vi "PCSMain.panel.vi"(0 "object ref":refnum<vi>, 5 "error in (no error)":errorcluster) -> (19 "error out":errorcluster)   [LabVIEW 2014, in "PCSMain.lvlib"]
doc: "This is just an example for a GUI thread.\n\nLicense Agreement for this software:\n\nCopyright (C)\nGesellschaft für Schwerionenforschung, GSI\nPlanckstr. 1\n64291 Darmstadt\nGermany\n\nContact: D.Beck@gsi.de \n\nThis program is free software; you can redistribute it and/or modify it under the terms of the GNU General Public License as published by the Free Software Foundation; either version 2 of the license, or (at your option) any later version.\n\nThis program is distributed in the hope that it will be useful, but WITHOUT ANYW ARRANTY; without even the implied warranty of MERCHANTABILITY or FITNESS FOR A PARTICULAR PURPOSE. See the GNU General License for more details (http://www.gnu.org).\n\nGesellschaft für Schwerionenforschung, GSI\nPlanckstr. 1, 64291 Darmstadt, Germany\nFor all questions and ideas contact: M.Richter@gsi.de, H.Brand@gsi.de or D.Beck@gsi.de.\nLast update: 18-DEC-2002"
uses:
  PCSMain.lvlib
  CSCore/CSObj/CSObj.lvlib
  PH_Common/PH_Common.lvlib
panel:
  in  "VISA":bool
  in  "Powermeter Statistician":bool
  in  "Powermeter List":bool
  in  "SHS Anal Statistician":bool
  in  "SHS Analyzer":bool
  in  "SHS Analysis Calibrator":bool
  in  "Remote Desktop Connection":bool
  in  "Minimize":bool
  in  "Beckhoff Watch Dog":bool
  in  "Countdown":bool
  in  "Seq Watch":bool
  in  "Vacuum Controllers":bool
  in  "SSAC":bool
  in  "Switch List":bool
  in  "BB List":bool
  in  "Spectrometer":bool
  in  "Z6 Beamline":bool
  in  "6P List":bool
  in  "Scopes":bool
  in  "Current Meas":bool
  in  "Calorimeter":bool
  in  "Cam List":bool
  in  "PCS System Indicator":bool caption="PCS"
  in  "Fast CoG":bool
  in  "Image Statistician":bool
  in  "Powermeter":bool
  in  "DataViewer":bool
  in  "Beamline":bool
  out "stopped":bool
  in  "BlackBoxes":bool
  in  "Operators":bool
  in  "Calibrator":bool
  in  "GateDelayGens":bool
  in  "Switch GUIs":bool
  in  "Motion GUIs":bool
  in  "Cameras":bool
  in  "Sequencer":bool
  in  "Delete":bool
  out "loop counter":i32
  # "PCS"
  # "3.40"
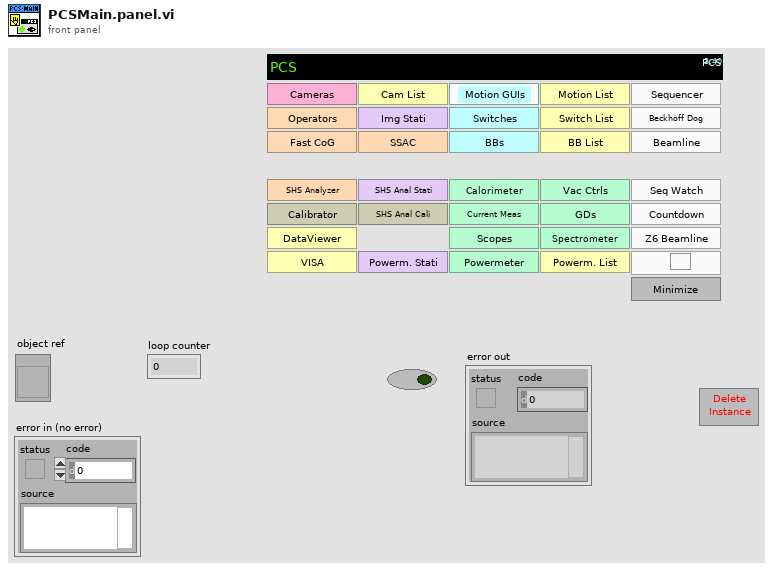
[diagram p1: front panel]
types:
  T1 = enum16{"None", "PCS Main", "Z6 Main", "PCS Beamline", "Z6 Beamline", "Image Statistician", "Powermeter Statistician", "SHS Anal Statistician", "Image Center of Gravity", "Image Calibrator", "SHS Analysis Calibrator"}
  T2 = enum16{"None", "PCS Main", "Z6 Main", "PCS Beamline", "Z6 Beamline", "Image Statistician", "Powermeter Statistician", "SHS Anal Statistician", "Image Center of Gravity", "Image Calibrator", "SHS Analysis Calibrator", "Cam List", "Powermeterlist", "6P List", "BB List", "Switch List", "Sequence Watch"}
  T3 = typedef "PCSMain.lvlib/PCSMain.i attribute.ctl" = cluster{"System Objects":cluster{"Spectrometer Objects":string[], "Camera Objects":string[], "Image Operator Objects":string[], "Gate- and Delaygenerators":string[], "Current Meas Objects":string[], "Calorimeter Objects":string[], "Powermeter Objects":string[], "SSAC Objects":string[], "Vacuum Control Objects":string[], "Countdown Counter Objects":string[], "Beckhoff Watchdog Objects":string[], "SHS Analyzer Objects":string[]}, "Local Objects":cluster{"Spectrometer Objects":string[], "Camera Objects":string[], "Image Operator Objects":string[], "Gate- and Delaygenerators":string[], "Current Meas Objects":string[], "Calorimeter Objects":string[], "Powermeter Objects":string[], "SSAC Objects":string[], "Vacuum Control Objects":string[], "Countdown Counter Objects":string[], "Beckhoff Watchdog Objects":string[], "SHS Analyzer Objects":string[]}, "Systems on same node":string[], "Data Viewer visible?":bool, "Running Objects":cluster{"Operators":bool, "SHS Analyzers":bool}, "Cam Instance System ID":string, "Black Box Objects":string[], "Switch Objects":string[], "Motion GUI Objects":string[], "Osci Objects":string[]}
  T4 = enum16{"PCS", "Laser", "Vision", "PP", "Special", "Beckhoff"}
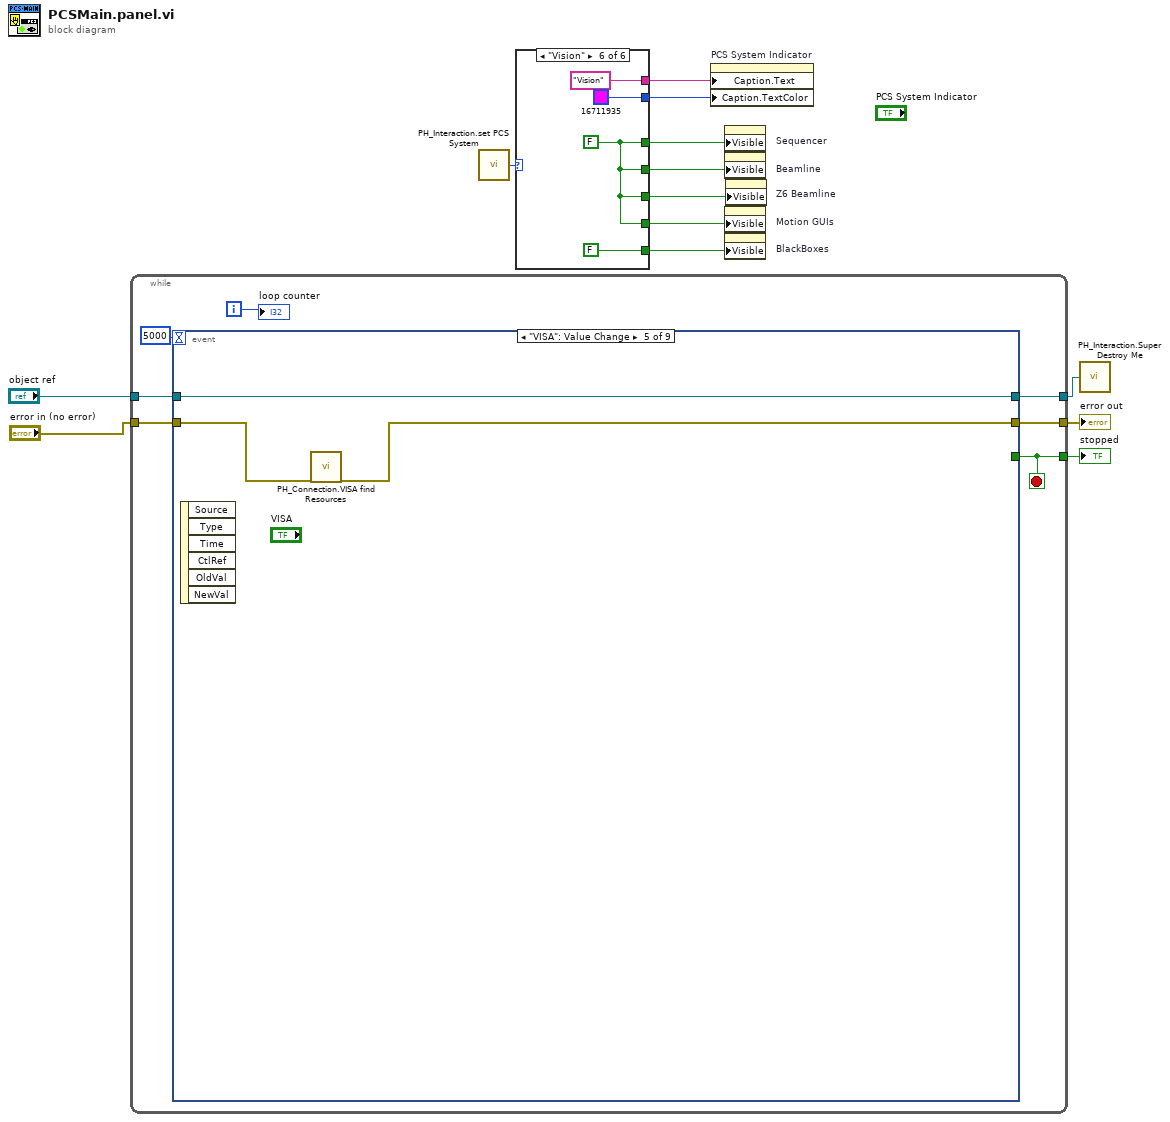
[diagram p0: block diagram]
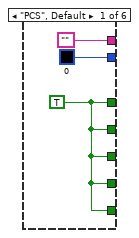
[diagram p2: hidden frame]
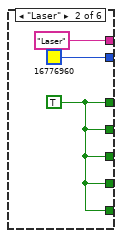
[diagram p3: hidden frame]
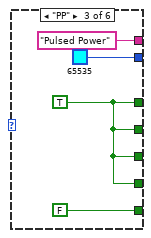
[diagram p4: hidden frame]
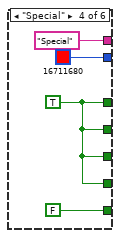
[diagram p5: hidden frame]
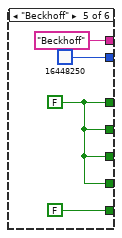
[diagram p6: hidden frame]
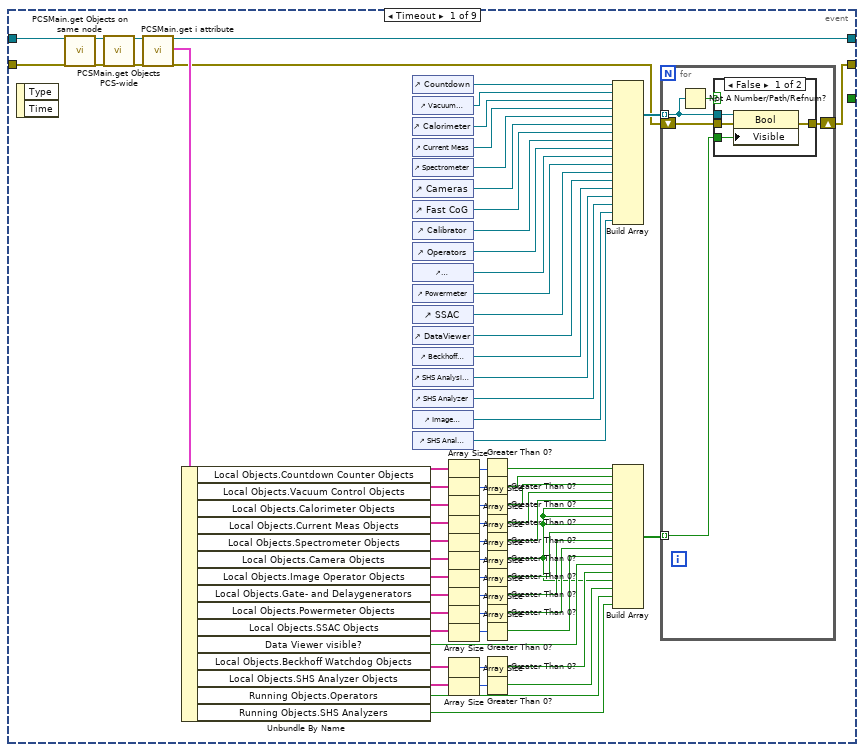
[diagram p7: hidden frame]
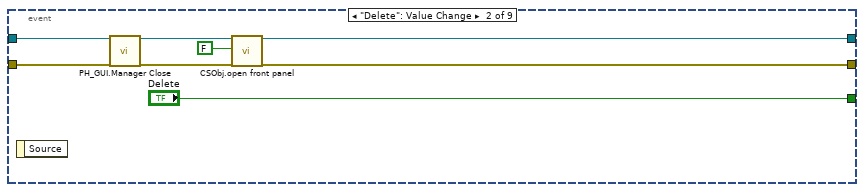
[diagram p9: hidden frame]
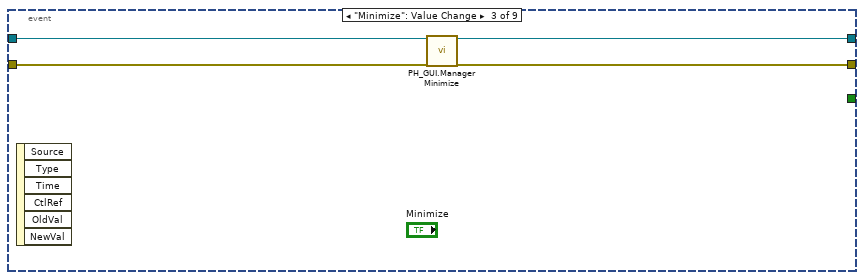
[diagram p10: hidden frame]
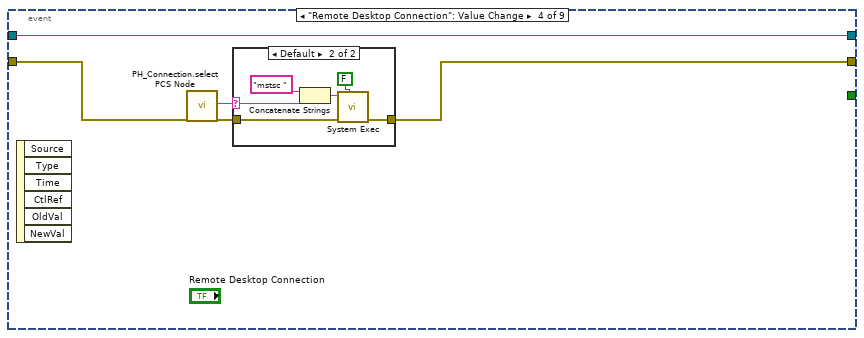
[diagram p11: hidden frame]
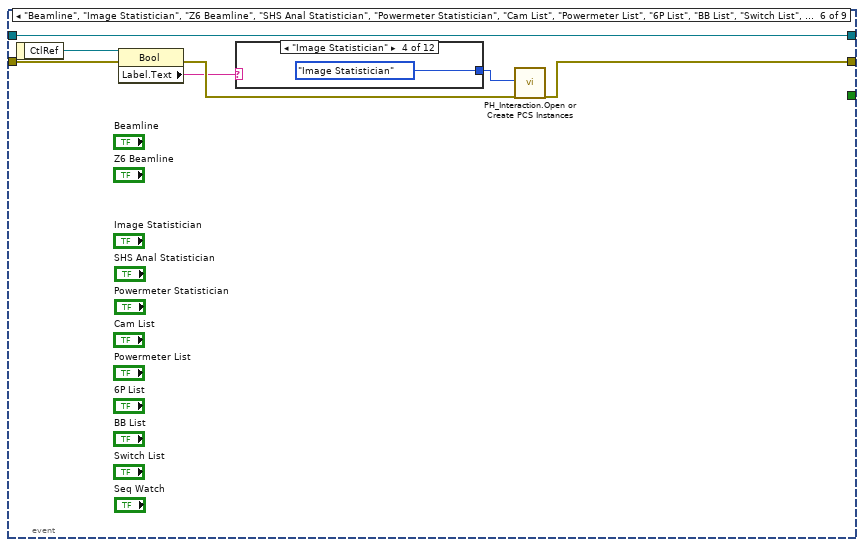
[diagram p13: hidden frame]
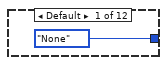
[diagram p14: hidden frame]
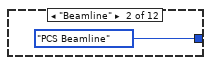
[diagram p15: hidden frame]
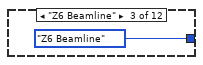
[diagram p16: hidden frame]
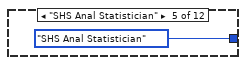
[diagram p17: hidden frame]
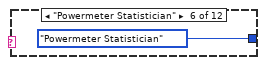
[diagram p18: hidden frame]
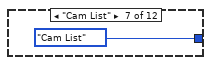
[diagram p19: hidden frame]
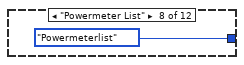
[diagram p20: hidden frame]
diagram:
  n1 = while {
    tunnel: "object ref" -> [w16]
    tunnel: [w15] -> w11
    tunnel: [w19] -> w12
    tunnel: "error in (no error)" -> [w18]
    tunnel: [w17] -> w13
    i -> [w20]
    stop <- w17 stop-if-true
    n2 = event shown="[4] \"VISA\": Value Change" {
      selector: _ -> [_ _ _ _ _ _ _ _ _]
      dyn-events: _ -> [_ _ _ _ _ _ _ _ _]
      timeout: 5000 -> [_ _ _ _ _ _ _ _ _]
      tunnel: w16 -> [w88 w105 w111 w115 w126 w130 w151 w171 w236]
      tunnel: [_ "Delete" _ _ _ _ _ _ _] -> w17
      tunnel: [w63 w104 w108 w113 w124 w133 w156 w169 w234] -> w19
      tunnel: w18 -> [w89 w101 w110 w116 w125 w131 w154 w170 w233]
      tunnel: [w62 w103 w109 w115 w126 w130 w150 w161 w235] -> w15
      event Timeout {
        n3 = event-data() -> ()  [unwired: 1 in, 2 out]
        n4 = call "PCSMain.get Objects on same node.vi"("i ref in"=w88, "error in (no error)"=w89) -> ("i ref out"=w24:refnum<vi>, "error out"=w22:errorcluster)  [unwired: 16 in]
        n5 = call "PCSMain.get Objects PCS-wide.vi"("i ref in"=w24, "error in (no error)"=w22) -> ("i ref out"=w23:refnum<vi>, "error out"=w21:errorcluster)  [unwired: 16 in]
        n6 = call "PCSMain.get i attribute.vi"("i ref in"=w23, "error in (no error)"=w21) -> ("i ref out"=w62:refnum<vi>, "i attribute"=w87:T3, "error out"=w64:errorcluster)  [unwired: 15 in]
        n7 = Unbundle By Name(w87) -> ("Local Objects.Countdown Counter Objects"=w44:string[], "Local Objects.Vacuum Control Objects"=w48:string[], "Local Objects.Calorimeter Objects"=w83:string[], "Local Objects.Current Meas Objects"=w76:string[], "Local Objects.Spectrometer Objects"=w74:string[], "Local Objects.Camera Objects"=w72:string[], "Local Objects.Image Operator Objects"=w71:string[], "Local Objects.Gate- and Delaygenerators"=w69:string[], "Local Objects.Powermeter Objects"=w67:string[], "Local Objects.SSAC Objects"=w39:string[], "Data Viewer visible?"=w50:bool, "Local Objects.Beckhoff Watchdog Objects"=w41:string[], "Local Objects.SHS Analyzer Objects"=w31:string[], "Running Objects.Operators"=w26:bool, "Running Objects.SHS Analyzers"=w25:bool)
        n8 = control-ref of="Countdown"() -> (w45:refnum<vi>)
        n9 = control-ref of="Vacuum Controllers"() -> (w49:refnum<vi>)
        n10 = control-ref of="Calorimeter"() -> (w61:refnum<vi>)
        n11 = control-ref of="Current Meas"() -> (w60:refnum<vi>)
        n12 = control-ref of="Spectrometer"() -> (w59:refnum<vi>)
        n13 = control-ref of="Cameras"() -> (w58:refnum<vi>)
        n14 = control-ref of="Fast CoG"() -> (w54:refnum<vi>)
        n15 = control-ref of="Calibrator"() -> (w53:refnum<vi>)
        n16 = control-ref of="Operators"() -> (w57:refnum<vi>)
        n17 = control-ref of="GateDelayGens"() -> (w56:refnum<vi>)
        n18 = control-ref of="Powermeter"() -> (w55:refnum<vi>)
        n19 = control-ref of="SSAC"() -> (w52:refnum<vi>)
        n20 = control-ref of="DataViewer"() -> (w51:refnum<vi>)
        n21 = control-ref of="Beckhoff Watch Dog"() -> (w36:refnum<vi>)
        n22 = control-ref of="SHS Analysis Calibrator"() -> (w34:refnum<vi>)
        n23 = control-ref of="SHS Analyzer"() -> (w29:refnum<vi>)
        n24 = control-ref of="Image Statistician"() -> (w28:refnum<vi>)
        n25 = control-ref of="SHS Anal Statistician"() -> (w27:refnum<vi>)
        n26 = Array Size(array=w44) -> (size(s)=w42:i32)
        n27 = Array Size(array=w48) -> (size(s)=w46:i32)
        n28 = Array Size(array=w83) -> (size(s)=w84:i32)
        n29 = Array Size(array=w76) -> (size(s)=w81:i32)
        n30 = Array Size(array=w74) -> (size(s)=w80:i32)
        n31 = Array Size(array=w72) -> (size(s)=w79:i32)
        n32 = Array Size(array=w71) -> (size(s)=w78:i32)
        n33 = Array Size(array=w69) -> (size(s)=w77:i32)
        n34 = Array Size(array=w67) -> (size(s)=w65:i32)
        n35 = Array Size(array=w39) -> (size(s)=w38:i32)
        n36 = Array Size(array=w41) -> (size(s)=w40:i32)
        n37 = Array Size(array=w31) -> (size(s)=w32:i32)
        n38 = Greater Than 0?(x=w42) -> (x > 0?=w43:bool)
        n39 = Greater Than 0?(x=w46) -> (x > 0?=w47:bool)
        n40 = Greater Than 0?(x=w84) -> (x > 0?=w82:bool)
        n41 = Greater Than 0?(x=w81) -> (x > 0?=w75:bool)
        n42 = Greater Than 0?(x=w80) -> (x > 0?=w73:bool)
        n43 = Greater Than 0?(x=w79) -> (x > 0?=w33:bool)
        n44 = Greater Than 0?(x=w78) -> (x > 0?=w70:bool)
        n45 = Greater Than 0?(x=w77) -> (x > 0?=w68:bool)
        n46 = Greater Than 0?(x=w65) -> (x > 0?=w66:bool)
        n47 = Greater Than 0?(x=w38) -> (x > 0?=w37:bool)
        n48 = Greater Than 0?(x=w40) -> (x > 0?=w35:bool)
        n49 = Greater Than 0?(x=w32) -> (x > 0?=w30:bool)
        n50 = Build Array(w45, w49, w61, w60, w59, w58, w54, w53, w57, w56, w55, w52, w51, w36, w34, w29, w28, w27) -> (w86:refnum<vi>[])
        n51 = Build Array(w43, w47, w82, w75, w73, w33, w33, w33, w70, w68, w66, w37, w50, w35, w33, w30, w26, w25) -> (w85:bool[])
        n52 = for {
          tunnel: w85 -> [w90] mode=indexing
          tunnel: w86 -> [w93] mode=indexing
          shift-right: [w92] -> w63
          shift-left: w64 -> [w91]
          n53 = Not A Number/Path/Refnum?(number/path/refnum=w93) -> (NaN/Path/Refnum?=w94:bool)
          n54 = case shown="False" w94 {
            tunnel: w90 -> [w98 _]
            tunnel: w93 -> [w97 _]
            tunnel: w91 -> [w96 w99]
            tunnel: [w95 w99] -> w92
            frame False {
              n55 = property class="Bool"(reference=w97, error in=w96, "Visible"=w98) -> (error out=w95:errorcluster)  [unwired: 1 out]
            }
            frame True {
            }
          }
        }
      }
      event "Delete": Value Change {
        n56 = event-data() -> ()  [unwired: 1 in, 1 out]
        n57 = call "PH_GUI.Manager Close.vi"("i ref in"=w105, "error in"=w101) -> ("i ref out"=w102:refnum<vi>, "error out"=w100:errorcluster)  [unwired: 16 in]
        n58 = call "CSObj.open front panel.vi"("i ref in"=w102, "frontPanelOpen"=FALSE ("front panel open"), "error in (no error)"=w100) -> ("i ref out"=w103:refnum<vi>, "error out"=w104:errorcluster)  [unwired: 15 in]
      }
      event "Minimize": Value Change {
        n59 = event-data() -> ()  [unwired: 1 in, 6 out]
        n60 = call "PH_GUI.Manager Minimize.vi"("i ref in"=w111, "error in"=w110) -> ("i ref out"=w109:refnum<vi>, "error out"=w108:errorcluster)  [unwired: 16 in]
      }
      event "Remote Desktop Connection": Value Change {
        n61 = event-data() -> ()  [unwired: 1 in, 6 out]
        n62 = call "PH_Connection.select PCS Node.vi"("error in"=w116) -> ("string out"=w112:string, "error out"=w114:errorcluster)  [unwired: 17 in]
        n63 = case shown="Default" w112 {
          selector: w112 -> [_ w118]
          tunnel: w114 -> [w117 w120]
          tunnel: [w117 w119] -> w113
          frame "", "N/A" {
          }
          frame Default {
            n64 = Concatenate Strings("mstsc " ("command line"), w118) -> (w122:string)
            n65 = call <vilib>:"System Exec.vi"("wait until completion? (T)"=FALSE, "error in (no error)"=w120, "command line"=w122) -> ("error out"=w119:errorcluster)  [unwired: 5 in, 3 out]
          }
        }
      }
      event "VISA": Value Change {
        n66 = event-data() -> ()  [unwired: 1 in, 6 out]
        n67 = call "PH_Connection.VISA find Resources.vi"("error in"=w125) -> ("error out"=w124:errorcluster)  [unwired: 17 in, 1 out]
      }
      event "Beamline", "Image Statistician", "Z6 Beamline", "SHS Anal Statistician", "Powermeter Statistician", "Cam List", "Powermeter List", "6P List", "BB List", "Switch List", "Seq Watch": Value Change {
        n68 = event-data() -> ("CtlRef"=w132:refnum<vi>)  [unwired: 1 in]
        n69 = property class="Bool"(reference=w132, error in=w131) -> (error out=w129:errorcluster, "Label.Text"=w128:string)  [unwired: 1 out]
        n70 = case shown="\"Image Statistician\"" w128 {
          tunnel: [T1."None" ("Instance to create or open") T1."PCS Beamline" ("Instance to create or open") T1."Z6 Beamline" ("Instance to create or open") T1."Image Statistician" ("Instance to create or open") T1."SHS Anal Statistician" ("Instance to create or open") T1."Powermeter Statistician" ("Instance to create or open") T2."Cam List" ("Instance to create or open") T2."Powermeterlist" ("Instance to create or open") T2."6P List" ("Instance to create or open") T2."BB List" ("Instance to create or open") T2."Switch List" ("Instance to create or open") T2."Sequence Watch" ("Instance to create or open")] -> w127
          frame Default {
          }
          frame "Beamline" {
          }
          frame "Z6 Beamline" {
          }
          frame "Image Statistician" {
          }
          frame "SHS Anal Statistician" {
          }
          frame "Powermeter Statistician" {
          }
          frame "Cam List" {
          }
          frame "Powermeter List" {
          }
          frame "6P List" {
          }
          frame "BB List" {
          }
          frame "Switch List" {
          }
          frame "Seq Watch" {
          }
        }
        n71 = call "PH_Interaction.Open or Create PCS Instances.vi"("Instance to create or open"=w127, "error IO"=w129) -> ("error out"=w133:errorcluster)  [unwired: 17 in]
      }
      event "Calibrator", "SHS Analysis Calibrator", "Fast CoG": Value Change {
        n72 = event-data() -> ("CtlRef"=w155:refnum<vi>)  [unwired: 1 in]
        n73 = property class="Bool"(reference=w155, error in=w154) -> (error out=w153:errorcluster, "Label.Text"=w146:string)  [unwired: 1 out]
        n74 = call "PCSMain.get i attribute.vi"("i ref in"=w151, "error in (no error)"=w153) -> ("i ref out"=w150:refnum<vi>, "i attribute"=w149:T3, "error out"=w152:errorcluster)  [unwired: 15 in]
        n75 = case shown="\"SHS Analysis Calibrator\"" w146 {
          tunnel: [T1."None" ("Instance to create or open") T1."Image Calibrator" ("Instance to create or open") T1."SHS Analysis Calibrator" ("Instance to create or open") T1."Image Center of Gravity" ("Instance to create or open")] -> w147
          frame Default {
          }
          frame "Calibrator" {
          }
          frame "SHS Analysis Calibrator" {
          }
          frame "Fast CoG" {
          }
        }
        n76 = Unbundle By Name(w149) -> ("Cam Instance System ID"=w148:string)
        n77 = call "PH_Interaction.Open or Create PCS Instances.vi"("System ID (N/A)"=w148, "Instance to create or open"=w147, "error IO"=w152) -> ("error out"=w156:errorcluster)  [unwired: 16 in]
      }
      event "Spectrometer", "Cameras", "Operators", "GateDelayGens", "Current Meas", "Calorimeter", "Powermeter", "SSAC", "Vacuum Controllers", "Beckhoff Watch Dog", "SHS Analyzer", "Switch GUIs", "BlackBoxes", "Motion GUIs", "Scopes": Value Change {
        n78 = event-data() -> ("CtlRef"=w167:refnum<vi>)  [unwired: 1 in]
        n79 = property class="Bool"(reference=w167) -> ("Label.Text"=w165:string)  [unwired: 1 in, 2 out]
        n80 = call "PCSMain.get i attribute.vi"("i ref in"=w171, "error in (no error)"=w170) -> ("i ref out"=w162:refnum<vi>, "i attribute"=w166:T3, "error out"=w168:errorcluster)  [unwired: 15 in]
        n81 = case shown="\"Spectrometer\"" w165 {
          tunnel: w166 -> [_ w179 w182 w185 w188 w191 w194 w197 w200 w203 w206 w209 w212 w215 w218 w221]
          tunnel: [string[] [] ("Spectrometer Objects") w178 w180 w183 w186 w189 w193 w196 w199 w202 w205 w208 w211 w214 w217 w220] -> w163
          tunnel: ["N/A" ("Caption.Text") "Spectrometer" ("Caption.Text") "Switch GUIs" ("Caption.Text") "Black Boxes" ("Caption.Text") "Motion GUIs" ("Caption.Text") "Oscilloscopes" ("Caption.Text") "Cameras" ("Caption.Text") "Image Operators" ("Caption.Text") "SHS Analyzers" ("Caption.Text") "Gate and Delay Generators" ("Caption.Text") "Current Measurement" ("Caption.Text") "Calorimeter" ("Caption.Text") "Powermeter" ("Caption.Text") "SSAC" ("Caption.Text") "Vacuum Controller" ("Caption.Text") "Beckhoff Watchdog" ("Caption.Text")] -> w164
          frame Default {
          }
          frame "Spectrometer" {
            n82 = Unbundle By Name(w179) -> ("Local Objects.Spectrometer Objects"=w178:string[])
          }
          frame "Switch GUIs" {
            n83 = Unbundle By Name(w182) -> ("Switch Objects"=w180:string[])
          }
          frame "BlackBoxes" {
            n84 = Unbundle By Name(w185) -> ("Black Box Objects"=w183:string[])
          }
          frame "Motion GUIs" {
            n85 = Unbundle By Name(w188) -> ("Motion GUI Objects"=w186:string[])
          }
          frame "Scopes" {
            n86 = Unbundle By Name(w191) -> ("Osci Objects"=w189:string[])
          }
          frame "Cameras" {
            n87 = Unbundle By Name(w194) -> ("Local Objects.Camera Objects"=w193:string[])
          }
          frame "Operators" {
            n88 = Unbundle By Name(w197) -> ("Local Objects.Image Operator Objects"=w196:string[])
          }
          frame "SHS Analyzer" {
            n89 = Unbundle By Name(w200) -> ("Local Objects.SHS Analyzer Objects"=w199:string[])
          }
          frame "GateDelayGens" {
            n90 = Unbundle By Name(w203) -> ("Local Objects.Gate- and Delaygenerators"=w202:string[])
          }
          frame "Current Meas" {
            n91 = Unbundle By Name(w206) -> ("Local Objects.Current Meas Objects"=w205:string[])
          }
          frame "Calorimeter" {
            n92 = Unbundle By Name(w209) -> ("Local Objects.Calorimeter Objects"=w208:string[])
          }
          frame "Powermeter" {
            n93 = Unbundle By Name(w212) -> ("Local Objects.Powermeter Objects"=w211:string[])
          }
          frame "SSAC" {
            n94 = Unbundle By Name(w215) -> ("Local Objects.SSAC Objects"=w214:string[])
          }
          frame "Vacuum Controllers" {
            n95 = Unbundle By Name(w218) -> ("Local Objects.Vacuum Control Objects"=w217:string[])
          }
          frame "Beckhoff Watch Dog" {
            n96 = Unbundle By Name(w221) -> ("Local Objects.Beckhoff Watchdog Objects"=w220:string[])
          }
        }
        n97 = call "PH_Strings.select string from array.vi"("String Array in"=w163, "Caption.Text"=w164, "error in (no error)"=w168) -> ("string out"=w174:string, "index"=w172:i32, "error out"=w173:errorcluster)  [unwired: 14 in]
        n98 = case shown="Default" w172 {
          tunnel: w173 -> [w223 w228]
          tunnel: [w223 w227] -> w169
          tunnel: w174 -> [_ w226]
          tunnel: w162 -> [w222 w224]
          tunnel: [w222 w225] -> w161
          frame -1 {
          }
          frame Default {
            n99 = call "PH_Interaction.Open or Create Singleton Instance.vi"("i ref in"=w224, "Instance to create or to open"=w226, "error IO"=w228) -> ("i ref out"=w225:refnum<vi>, "error out"=w227:errorcluster)  [unwired: 15 in]
          }
        }
      }
      event "DataViewer", "Countdown", "Sequencer": Value Change {
        n100 = event-data() -> ("CtlRef"=w231:refnum<vi>)  [unwired: 1 in]
        n101 = property class="Bool"(reference=w231, error in=w233) -> (error out=w232:errorcluster, "Label.Text"=w230:string)  [unwired: 1 out]
        n102 = case shown="\"Countdown\"" w230 {
          tunnel: ["N/A" "Data_Viewer" "PHELIX_Sequencer_1" "Countdown"] -> w229
          frame Default {
          }
          frame "DataViewer" {
          }
          frame "Sequencer" {
          }
          frame "Countdown" {
          }
        }
        n103 = call "PH_Interaction.Open or Create Singleton Instance.vi"("i ref in"=w236, "Instance to create or to open"=w229, "error IO"=w232) -> ("i ref out"=w235:refnum<vi>, "error out"=w234:errorcluster)  [unwired: 15 in]
      }
    }
    "loop counter" <- w20
  }
  "error out" <- w12
  "stopped" <- w13
  n104 = call "PH_Interaction.set PCS System.vi"() -> ("Enum"=w10:T4)  [unwired: 1 in]
  n105 = case shown="\"Vision\"" w10 {
    tunnel: ["" "Laser" "Pulsed Power" "Special" "Beckhoff" "Vision"] -> w9
    tunnel: [w242 w245 w249 w253 w257 w261] -> w8
    tunnel: [w242 w245 w249 w253 w257 w261] -> w7
    tunnel: [w242 w245 w249 w253 w257 w261] -> w6
    tunnel: [w242 w245 FALSE FALSE FALSE FALSE] -> w5
    tunnel: [w242 w245 w249 w253 w257 w261] -> w4
    tunnel: [u32 0 ("Color Box") u32 16776960 ("Color Box") u32 65535 ("Color Box") u32 16711680 ("Color Box") u32 16448250 ("Color Box") u32 16711935 ("Color Box")] -> w1
    frame "PCS", Default {
      w242 = TRUE
    }
    frame "Laser" {
      w245 = TRUE
    }
    frame "PP" {
      w249 = TRUE
    }
    frame "Special" {
      w253 = TRUE
    }
    frame "Beckhoff" {
      w257 = FALSE
    }
    frame "Vision" {
      w261 = FALSE
    }
  }
  n106 = property on="PCS System Indicator" class="Bool (strict)"("Caption.Text"=w9, "Caption.TextColor"=w1) -> ()  [unwired: 2 in, 2 out]
  n107 = property on="Sequencer" class="Bool"("Visible"=w8) -> ()  [unwired: 2 in, 2 out]
  n108 = property on="Beamline" class="Bool"("Visible"=w7) -> ()  [unwired: 2 in, 2 out]
  n109 = property on="Motion GUIs" class="Bool"("Visible"=w6) -> ()  [unwired: 2 in, 2 out]
  n110 = property on="BlackBoxes" class="Bool"("Visible"=w5) -> ()  [unwired: 2 in, 2 out]
  n111 = property on="Z6 Beamline" class="Bool"("Visible"=w4) -> ()  [unwired: 2 in, 2 out]
  n112 = call "PH_Interaction.Super Destroy Me.vi"("i ref out"=w11) -> ()
